vi "TDMS Find Max Run Matching Field.vi"(8 "error in (no error)":errorcluster, 9 "Property Value":string, 10 "Property Name":string, 11 "TDMS File Path":path) -> (0 "error out":errorcluster, 1 "Found?":bool, 2 "Run ID":string, 3 "TDMS File Path Out":path)   [LabVIEW 2011]
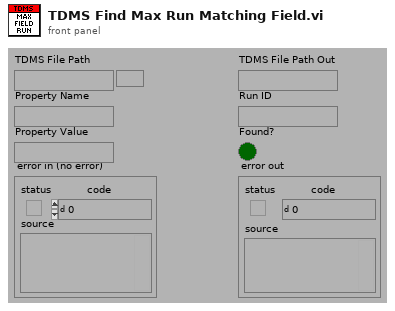
[diagram p1: front panel]
types:
  T1 = enum16{"open", "open or create", "create or replace", "create", "open (read-only)"}
  T2 = typedef "Connection Refnum.ctl" = cluster{"Environment Handle":i32, "Connection Handle":i32}
  T3 = typedef "Field Record.ctl" = cluster{"ixField":i32, "iSequenceOrder":i32, "sxFieldId":string, "sxSequenceId":string, "sDisplayName":string, "sValue":string, "sUnits":string, "nDataType":T4, "nNextItem":T5, "fSystem":bool, "fSystemValue":bool, "fRequired":bool, "fSetAtTest":bool, "fTestField":bool, "fDeleted":bool, "fIndexed":bool, "fFreeList":bool}
  T4 = typedef "Field DataTypes.ctl" = enum32{"text", "numeric", "list", "timestamp", "boolean"}
  T5 = typedef "Field NextItem.ctl" = enum32{"Reset", "Retain", "Auto-Increment"}
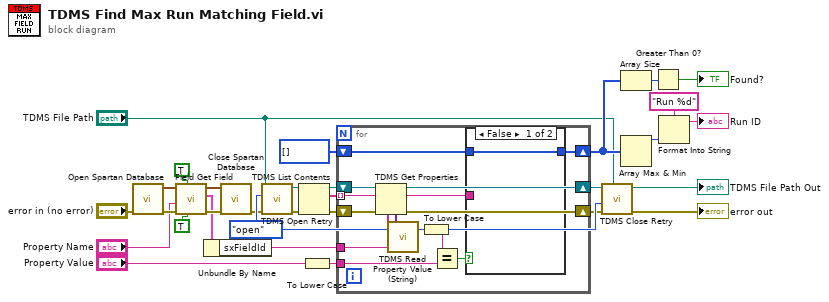
[diagram p0: block diagram]
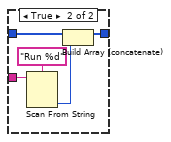
[diagram p2: hidden frame]
diagram:
  w30 = T1."open" ("operation (0:open)")
  n1 = call "Open Spartan Database.vi"("error in (no error)"="error in (no error)") -> ("error out"=w11:errorcluster, "Connection Refnum"=w10:T2)  [unwired: 9 in]
  n2 = call "Field Get Field.vi"("by sDisplayName? (f, by sFieldId)"=TRUE, "Include deleted? (F)"=TRUE, "error in (no error)"=w11, "sFieldId or sDisplayName (\"\")"="Property Name", "Connection Refnum"=w10) -> ("error out"=w8:errorcluster, "Field"=w3:T3, "Connection Refnum"=w9:T2)  [unwired: 3 in, 1 out]
  n3 = Unbundle By Name(w3) -> ("sxFieldId"=w1:string)
  n4 = call "Close Spartan Database.vi"("error in (no error)"=w8, "Connection Refnum"=w9) -> ("error out"=w6:errorcluster)  [unwired: 9 in]
  n5 = call "TDMS Open Retry.vi"("error in (no error)"=w6, "Operation (0:open)"=w30, "Path"="TDMS File Path") -> ("error out"=w29:errorcluster, "TDMS File Ref"=w27:refnum<k34>)  [unwired: 1 in, 6 out]
  n6 = TDMS List Contents(4:w29, 7:w27) -> (0:w28:errorcluster, 2:w25:string[], 3:w26:refnum<k34>)  [unwired: 1 in, 1 out]
  n7 = To Lower Case(string="Property Value") -> (all lower case string=w23:string)
  n8 = for {
    tunnel: w25 -> [w44] mode=indexing
    tunnel: w1 -> [w41]
    tunnel: w23 -> [w38]
    shift-right: [w34] -> w16
    shift-left: i32[] [] -> [w36]
    shift-right: [w33] -> w18
    shift-left: w28 -> [w46]
    shift-right: [w32] -> w19
    shift-left: w26 -> [w45]
    n9 = TDMS Get Properties(8:w46, 10:w44, 11:w45) -> (0:w33:errorcluster, 2:w35:string, 3:w32:refnum<k34>, 4:w43:variant[], 6:w42:string[])  [unwired: 3 in, 1 out]
    n10 = call "TDMS Read Property Value (String).vi"("Property Name"=w41, "Property Names"=w42, "Property Values"=w43) -> ("Property Value"=w40:string)  [unwired: 1 out]
    n11 = To Lower Case(string=w40) -> (all lower case string=w39:string)
    n12 = Equal?(x=w39, y=w38) -> (x = y?=w37:bool)
    n13 = case shown="False" w37 {
      tunnel: w36 -> [w47 w50]
      tunnel: w35 -> [_ w52]
      tunnel: [w47 w49] -> w34
      frame False {
      }
      frame True {
        n14 = Scan From String(format string="Run %d", input string=w52) -> (output 1=w48:i32)  [unwired: 3 in, 3 out]
        n15 = Build Array (concatenate)(w50, w48) -> (w49:i32[])
      }
    }
  }
  n16 = call "TDMS Close Retry.vi"("TDMS Path"="TDMS File Path", "error in (no error)"=w18, "Operation (0:open)"=w30, "TDMS File Ref"=w19) -> ("error out"=→"error out":errorcluster, "TDMS Path Out"=→"TDMS File Path Out":path)  [unwired: 1 in, 5 out]
  n17 = Array Size(array=w16) -> (size(s)=w15:i32)
  n18 = Array Max & Min(array=w16) -> (max value=w20:i32)  [unwired: 3 out]
  n19 = Greater Than 0?(x=w15) -> (x > 0?=→"Found?":bool)
  n20 = Format Into String(format string="Run %d", w20) -> (resulting string=→"Run ID":string)  [unwired: 2 in, 1 out]
